vi "loadLocalVI.vi"(8 "error in":errorcluster, 11 "fileName":string) -> (0 "error out":errorcluster, 3 "vi reference":refnum<vi>)   [LabVIEW 2010]
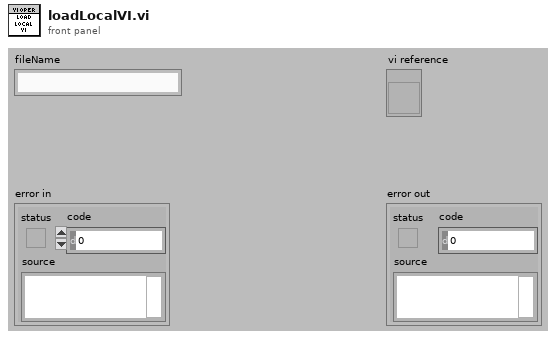
[diagram p1: front panel]
types:
  T1 = enum32{"Bad", "Idle", "Run top level", "Running"}
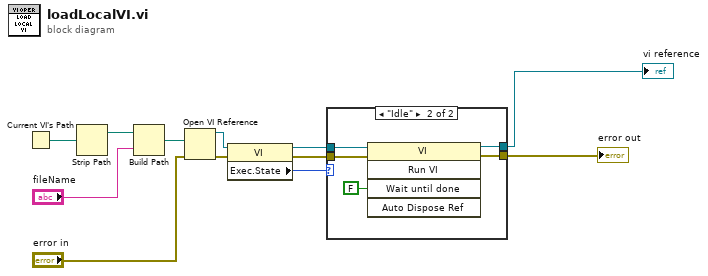
[diagram p0: block diagram]
diagram:
  n1 = Current VI's Path() -> (path=w12:path)
  n2 = Strip Path(path=w12) -> (stripped path=w11:path)  [unwired: 1 out]
  n3 = Build Path(base path=w11, name or relative path="fileName") -> (appended path=w10:path)
  n4 = Open VI Reference(vi path=w10, error in (no error)="error in") -> (vi reference=w8:refnum<vi>, error out=w9:errorcluster)  [unwired: 4 in]
  n5 = property class="VI"(reference=w8, error in=w9) -> (reference out=w5:refnum<vi>, error out=w6:errorcluster, "Exec.State"=w7:T1)
  n6 = case shown="\"Idle\"" w7 {
    tunnel: w6 -> [w14 w19]
    tunnel: w5 -> [w13 w18]
    tunnel: [w14 w16] -> w1
    tunnel: [w13 w15] -> w2
    frame "Bad", Default {
    }
    frame "Idle" {
      n7 = invoke class="VI" method="Run VI"(reference=w18, error in=w19, "Wait until done"=FALSE ("Wait Until Done")) -> (reference out=w15:refnum<vi>, error out=w16:errorcluster)  [unwired: 2 in, 3 out]
    }
  }
  "error out" <- w1
  "vi reference" <- w2
